vi "PID - Tool.vi"() -> ()   [LabVIEW 2019, in "Control Workspace Tool.lvlib"]
uses:
  Control Workspace Tool.lvlib
  NationalInstruments.VeriStand.SystemStorage
  Types/Tool State Variables.ctl
  Addon/Addon Shared/Types/Get Settings Message.ctl
  Addon/Addon Shared/Types/Gain Schedule.ctl
  <vilib>/NI VeriStand/Execution/Workspace/WorkspaceAPI.ctl
  <vilib>/NI VeriStand/Execution/Workspace/SystemStateRegEventRef.ctl
  <vilib>/NI VeriStand/Execution/Workspace/Target State Info.ctl
  <vilib>/NI VeriStand/Execution/Workspace/Target State.ctl
  <vilib>/NI VeriStand/Execution/Workspace/SystemStateEventRef.ctl
  <vilib>/NI/STM/TCP/TCP Connection Info.ctl
  <vilib>/NI/STM/SubVIs/MetaDataElement.ctl
  Types/UI Refs.ctl
  Workspace Objects/Types/UDP Streaming Command Cluster.ctl
  Workspace Objects/Types/UDP Streaming State.ctl
  Workspace Objects/Types/UI.Chart.Refs.ctl
  Addon/Addon Shared/Types/Update Parameters Message.ctl
  Addon/Addon Shared/SubVIs/Constants.vi
  <vilib>/NI VeriStand/Execution/Workspace/NI VeriStand - Set Single Channel Value.vi
  <vilib>/NI VeriStand/Execution/Workspace/NI VeriStand - Get Multiple Channel Values.vi
  NationalInstruments.VeriStand.SystemDefinitionAPI
  APIs/Host Automation API/Control Host Automation API.lvlib
  Addon/Addon Shared/Control Addon Shared.lvlib
  <vilib>/NI VeriStand/Execution/Workspace/NI_VS Workspace ExecutionAPI.lvlib
  <vilib>/NI/STM/NI STM.lvlib
  Workspace Shared/Control Workspace Shared.lvlib
  Workspace Objects/Control Workspace Object.lvlib
  NationalInstruments.VeriStand.ClientAPI
panel:
  in  "NIVS.Gateway IP Address":string
  out "Gain Scheduling Allowed?":bool
  in  "Revert":bool
  in  "Apply":bool
  out "Live Updates Allowed?":bool
  in  "PID Controller Name":u16(ring) items=["PID Controller", "PID Controller 1"]
  in  "PID Settings":i32(listbox)
  in  "NIVS.System Definition Root":refnum<k24>
  out "Device":string
  in  "NIVS.Workspace Event":refnum<event-registration>
  in  "Hold":bool
  out "Chart":waveform(dbl)[](graph)
  in  "Autoscale Y":bool=TRUE
  in  "Autoscale X":bool=TRUE
  in  "Manual Value":bool
  in  "Setpoint":dbl min=0.0 max=100.0
  in  "Manual Control":bool
  in  "Manual Output":dbl min=0.0 max=100.0
  in  "Revert Control Change":bool
  in  "Apply Control Change":bool
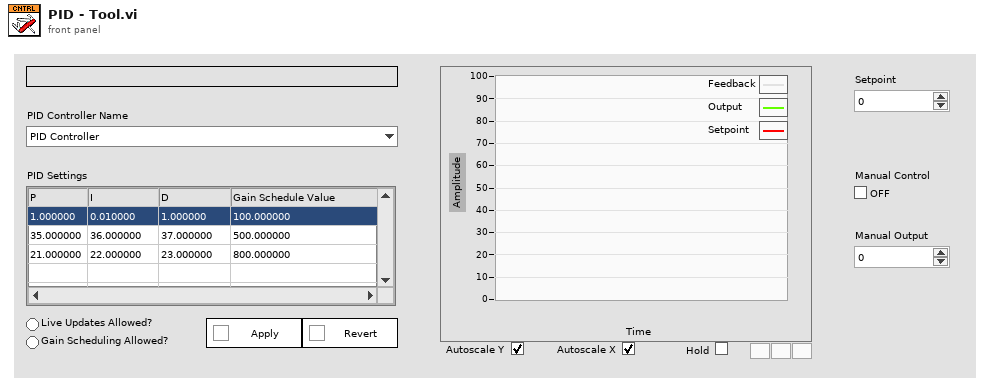
[diagram p1: front panel]
types:
  T1 = typedef "Control Workspace Tool.lvlib/Tool State Variables.ctl" = cluster{"CD Path":string, "CD IP":string, "Settings":T2, "NIVS.SysDefRoot":refnum<k24>, "NIVS.Workspace":T4, "NIVS.UserEvents":cluster{"NIVS.Workspace Event":refnum<event-registration>, "SystemChangeEventRef":T5}, "NIVS.SystemStateRefs":T6, "UI.PIDSettingsMenu":string[], "Comm Info":T7, "Addon.Connected?":bool, "UI.Refs":T9, "NIVS.SysDef":refnum<k24>, "Data.UDPChannels":string[], "Data.Found?":bool, "Data.PreviousValues":dbl[], "Data.SlowChannels":string[], "Data.PendingChange?":bool, "Data.UDPEngineQueue":refnum<queue>, "UI.Chart.Refs":T10, "Controller.SetpointRange":cluster{"Min":dbl, "Max":dbl}, "Controller.OutputRange":cluster{"Min":dbl, "Max":dbl}}
  T2 = typedef "Control Addon Shared.lvlib/Get Settings Message.ctl" = cluster{"Control Loop Names":string[], "Enable Live Updates":bool[], "Gain Schedule":T3[], "Enable Gain Scheduling":bool[]}
  T3 = typedef "Control Addon Shared.lvlib/Gain Schedule.ctl" = cluster{"Gain Schedule":cluster{"PID gains":cluster{"proportional gain (Kc)":dbl, "integral time (Ti, min)":dbl, "derivative time (Td, min)":dbl}, "max value":dbl}[]}
  T4 = typedef "NI_VS Workspace ExecutionAPI.lvlib/WorkspaceAPI.ctl" = refnum<k24>
  T5 = typedef "NI_VS Workspace ExecutionAPI.lvlib/SystemStateRegEventRef.ctl" = refnum<event-registration>
  T6 = typedef "NI_VS Workspace ExecutionAPI.lvlib/SystemStateEventRef.ctl" = cluster{"CustDatRef":refnum<user-event>, "EvtRef":refnum<k27>, "Target State User Event":refnum<user-event>}
  T7 = typedef "NI STM.lvlib/TCP Connection Info.ctl" = cluster{"connection ID":refnum<k5>, "meta data":T8[]}
  T8 = typedef "NI STM.lvlib/MetaDataElement.ctl" = string
  T9 = typedef "Control Workspace Tool.lvlib/UI Refs.ctl" = cluster{"Controller":refnum<vi>, "GainSettings":refnum<vi>, "Device":refnum<vi>, "GainSchedulingAllowed?":refnum<vi>, "LiveUpdatesAllowed?":refnum<vi>, "Revert":refnum<vi>, "Apply":refnum<vi>}
  T10 = typedef "Control Workspace Object.lvlib/UI.Chart.Refs.ctl" = cluster{"Chart":refnum<vi>, "Manual Value":refnum<vi>, "Manual Output":refnum<vi>, "Revert":refnum<vi>, "Apply":refnum<vi>, "Setpoint":refnum<vi>, "Autoscale X":refnum<vi>, "Autoscale Y":refnum<vi>, "Hold":refnum<vi>, "Manual Control":refnum<vi>}
  T11 = typedef "Control Workspace Object.lvlib/UDP Streaming Command Cluster.ctl" = cluster{"Action":T12, "Channels":string[]}
  T12 = typedef "Control Workspace Object.lvlib/UDP Streaming State.ctl" = enum8{"Idle", "Start Acq", "Run", "Stop Acq", "Exit"}
  T13 = typedef "Control Addon Shared.lvlib/Update Parameters Message.ctl" = cluster{"Control Loop":string, "Gain Schedule":cluster{"PID gains":cluster{"proportional gain (Kc)":dbl, "integral time (Ti, min)":dbl, "derivative time (Td, min)":dbl}, "max value":dbl}[]}
  T14 = cluster{"NIVS.Workspace Event":refnum<event-registration>, "SystemChangeEventRef":T5}
  T15 = typedef "LVPoint32TypeDef.ctl" = cluster{"Horizontal":i32, "Vertical":i32}
  T16 = cluster{"PID gains":cluster{"proportional gain (Kc)":dbl, "integral time (Ti, min)":dbl, "derivative time (Td, min)":dbl}, "max value":dbl}[]
  T17 = cluster{"proportional gain (Kc)":dbl, "integral time (Ti, min)":dbl, "derivative time (Td, min)":dbl}
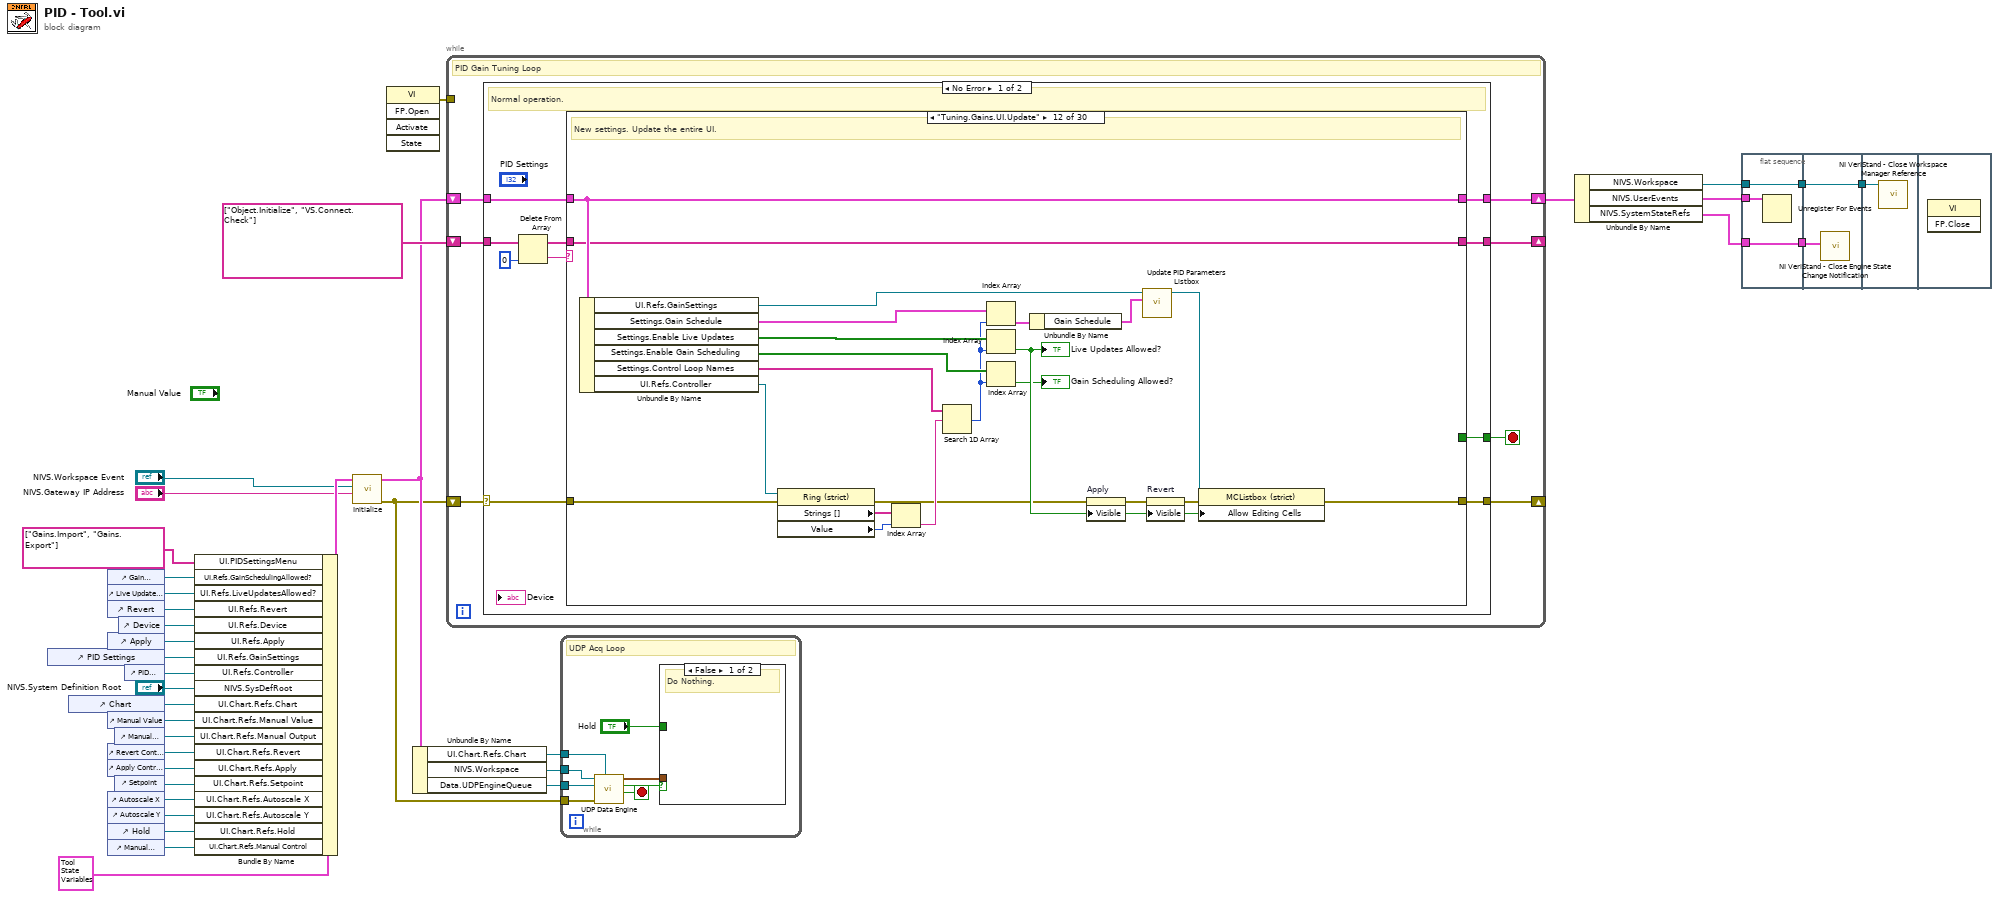
[diagram p0: block diagram]
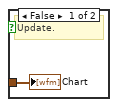
[diagram p3: hidden frame]
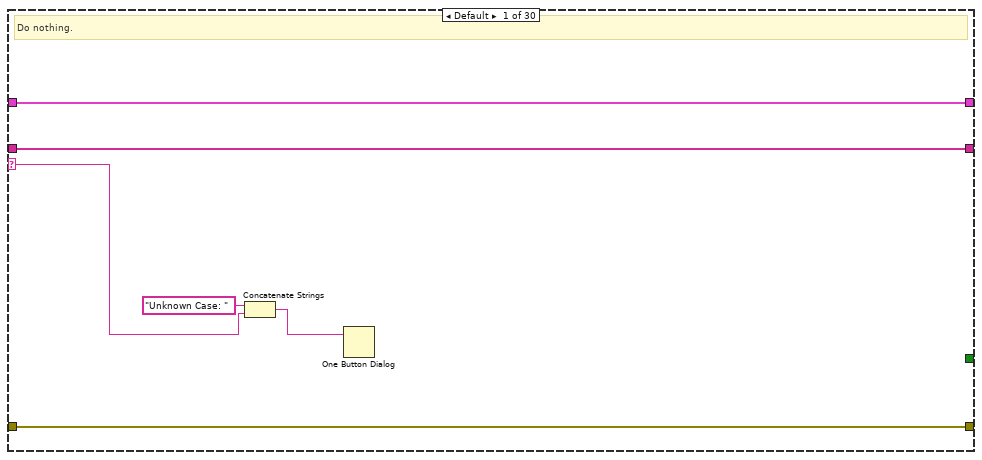
[diagram p4: hidden frame]
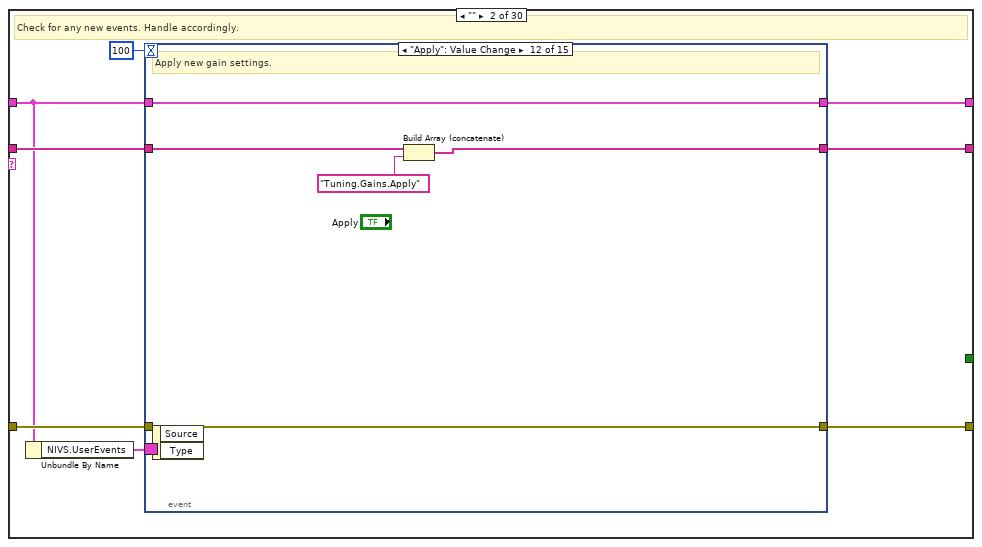
[diagram p5: hidden frame]
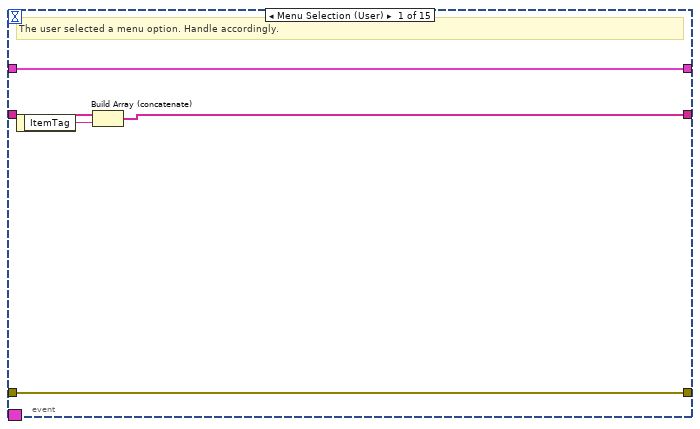
[diagram p6: hidden frame]
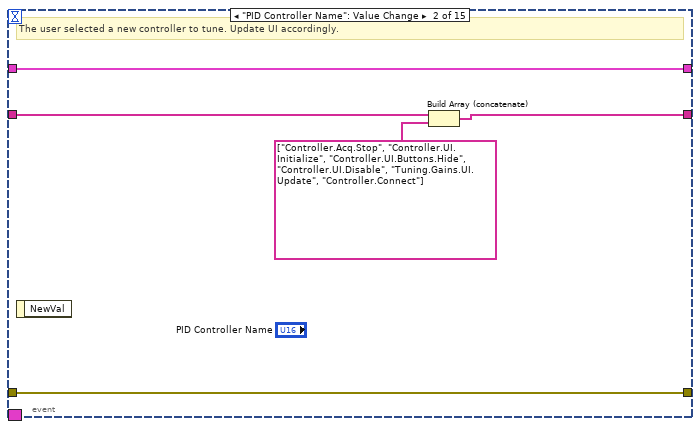
[diagram p7: hidden frame]
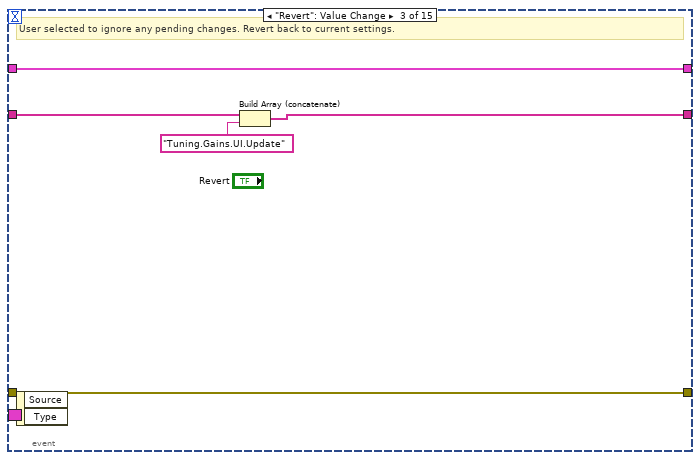
[diagram p8: hidden frame]
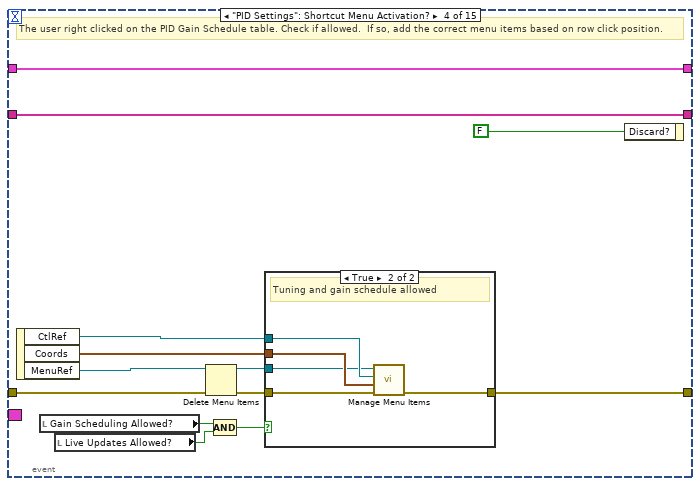
[diagram p9: hidden frame]
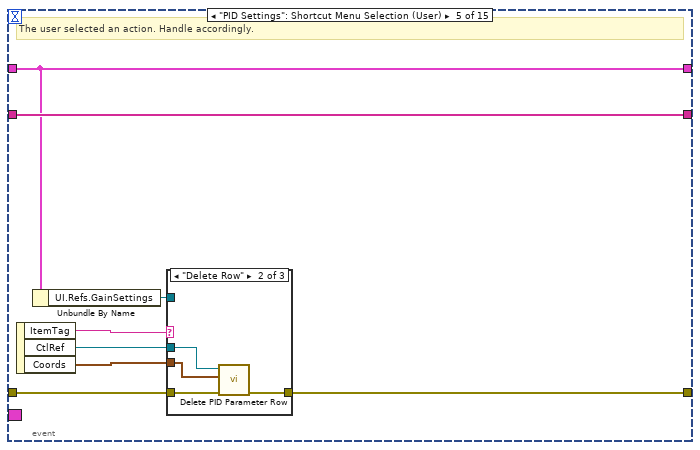
[diagram p11: hidden frame]
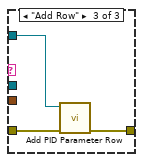
[diagram p13: hidden frame]
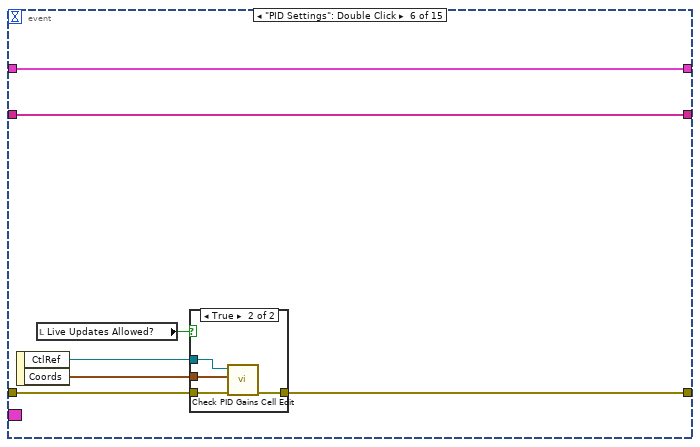
[diagram p14: hidden frame]
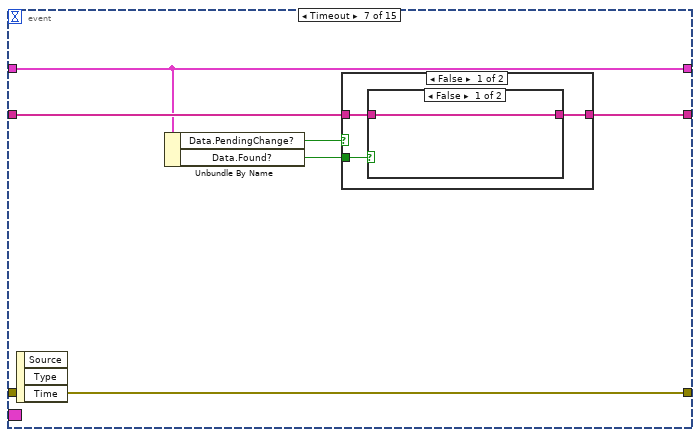
[diagram p16: hidden frame]
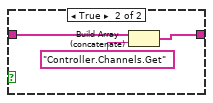
[diagram p17: hidden frame]
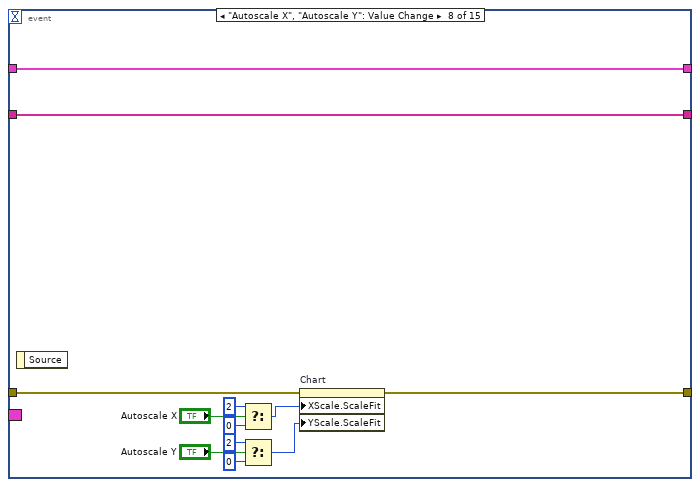
[diagram p19: hidden frame]
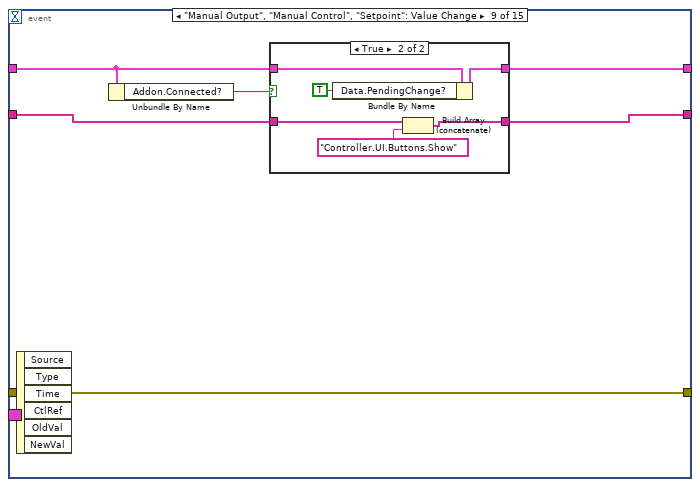
[diagram p20: hidden frame]
diagram:
  n1 = control-ref of="PID Settings"() -> (w32:refnum<vi>)
  n2 = control-ref of="Chart"() -> (w10:refnum<vi>)
  n3 = control-ref of="Gain Scheduling Allowed?"() -> (w24:refnum<vi>)
  n4 = control-ref of="Live Updates Allowed?"() -> (w23:refnum<vi>)
  n5 = control-ref of="Revert"() -> (w22:refnum<vi>)
  n6 = control-ref of="Apply"() -> (w21:refnum<vi>)
  n7 = control-ref of="Manual Value"() -> (w2:refnum<vi>)
  n8 = control-ref of="Revert Control Change"() -> (w9:refnum<vi>)
  n9 = control-ref of="Apply Control Change"() -> (w8:refnum<vi>)
  n10 = control-ref of="Autoscale X"() -> (w6:refnum<vi>)
  n11 = control-ref of="Autoscale Y"() -> (w5:refnum<vi>)
  n12 = control-ref of="Hold"() -> (w4:refnum<vi>)
  n13 = control-ref of="Manual Control"() -> (w3:refnum<vi>)
  n14 = control-ref of="Manual Output"() -> (w1:refnum<vi>)
  n15 = control-ref of="Setpoint"() -> (w7:refnum<vi>)
  n16 = control-ref of="Device"() -> (w20:refnum<vi>)
  n17 = control-ref of="PID Controller Name"() -> (w31:refnum<vi>)
  n18 = Bundle By Name(cluster=T1 {"CD Path"="", "CD IP"="", "Settings"={"Control Loop Names"=[], "Enable Live Updates"=[], "Gain Schedule"=[], "Enable Gain Scheduling"=[]}, "NIVS.SysDefRoot"=refnum, "NIVS.Workspace"=refnum, "NIVS.UserEvents"={"NIVS.Workspace Event"=refnum, "SystemChangeEventRef"=refnum}, "NIVS.SystemStateRefs"={"CustDatRef"=refnum, "EvtRef"=refnum, "Target State User Event"=refnum}, "UI.PIDSettingsMenu"=[], "Comm Info"={"connection ID"=refnum, "meta data"=[]}, "Addon.Connected?"=FALSE, "UI.Refs"={"Controller"=refnum, "GainSettings"=refnum, "Device"=refnum, "GainSchedulingAllowed?"=refnum, "LiveUpdatesAllowed?"=refnum, "Revert"=refnum, "Apply"=refnum}, "NIVS.SysDef"=refnum, "Data.UDPChannels"=[], "Data.Found?"=FALSE, "Data.PreviousValues"=[], "Data.SlowChannels"=[], "Data.PendingChange?"=FALSE, "Data.UDPEngineQueue"=refnum, "UI.Chart.Refs"={"Chart"=refnum, "Manual Value"=refnum, "Manual Output"=refnum, "Revert"=refnum, "Apply"=refnum, "Setpoint"=refnum, "Autoscale X"=refnum, "Autoscale Y"=refnum, "Hold"=refnum, "Manual Control"=refnum}, "Controller.SetpointRange"={"Min"=0.0, "Max"=0.0}, "Controller.OutputRange"={"Min"=0.0, "Max"=0.0}}, "UI.PIDSettingsMenu"=string[] ["Gains.Import", "Gains.Export"], "UI.Refs.GainSchedulingAllowed?"=w24, "UI.Refs.LiveUpdatesAllowed?"=w23, "UI.Refs.Revert"=w22, "UI.Refs.Device"=w20, "UI.Refs.Apply"=w21, "UI.Refs.GainSettings"=w32, "UI.Refs.Controller"=w31, "NIVS.SysDefRoot"="NIVS.System Definition Root", "UI.Chart.Refs.Chart"=w10, "UI.Chart.Refs.Manual Value"=w2, "UI.Chart.Refs.Manual Output"=w1, "UI.Chart.Refs.Revert"=w9, "UI.Chart.Refs.Apply"=w8, "UI.Chart.Refs.Setpoint"=w7, "UI.Chart.Refs.Autoscale X"=w6, "UI.Chart.Refs.Autoscale Y"=w5, "UI.Chart.Refs.Hold"=w4, "UI.Chart.Refs.Manual Control"=w3) -> (w15:T1)
  n19 = call "Initialize.vi"("NIVS.Gateway IP Address"="NIVS.Gateway IP Address", "NIVS.Workspace Event"="NIVS.Workspace Event", "State Variables"=w15) -> ("error out"=w11:errorcluster, "output cluster"=w12:T1)  [unwired: 7 in]
  n20 = invoke class="VI" method="FP.Open"() -> (error out=w36:errorcluster)  [unwired: 5 in, 4 out]
  n21 = Unbundle By Name(w12) -> ("UI.Chart.Refs.Chart"=w19:refnum<vi>, "NIVS.Workspace"=w18:T4, "Data.UDPEngineQueue"=w17:refnum<queue>)
  n22 = while {
    shift-right: [w42] -> w29
    shift-left: w12 -> [w43]
    shift-right: [w40] -> _
    shift-left: string[] ["Object.Initialize", "VS.Connect.Check"] -> [w41]
    tunnel: w36 -> [_]
    shift-right: [w39] -> _
    shift-left: w11 -> [w38]
    stop <- w44 stop-if-true
    # "PID Gain Tuning Loop"
    n23 = case shown="No Error" w38 {
      selector: w38 -> [w45 w764]
      tunnel: [w54 _] -> w44
      tunnel: w43 -> [w53 w766]
      tunnel: [w52 w766] -> w42
      tunnel: w41 -> [w51 w765]
      tunnel: [w47 w765] -> w40
      tunnel: [w46 w762] -> w39
      frame No Error {
        # "Normal operation."
        n24 = Delete From Array(array=w51, index=0) -> (deleted portion=w49:string, array with subset deleted=w48:string[])  [unwired: 1 in]
        n25 = case shown="\"Tuning.Gains.UI.Update\"" w49 {
          selector: w49 -> [w57 _ _ _ _ _ _ _ _ _ _ _ _ _ _ _ _ _ _ _ _ _ _ _ _ _ _ _ _ _]
          tunnel: [_ _ _ _ _ _ _ TRUE ("Discard?") _ _ _ _ _ _ _ _ _ _ _ _ _ _ _ _ _ _ _ _ _ _] -> w54
          tunnel: w53 -> [w59 w63 w223 w251 w268 w277 w296 w314 w319 w330 w338 w367 w370 w411 w440 w494 w512 w525 w538 w552 w573 w581 w625 w679 w702 w724 w732 w744 w752 w756]
          tunnel: [w59 w68 w224 w246 w268 w278 w297 w313 w319 w331 w339 w367 w370 w411 w448 w493 w512 w525 w538 w551 w573 w582 w626 w680 w703 w725 w733 w744 w747 w755] -> w52
          tunnel: w48 -> [w60 w67 w222 w245 w266 w280 w299 w316 w318 w337 w345 w346 w373 w413 w446 w490 w516 w527 w533 w555 w580 w599 w637 w691 w723 w731 w739 w745 w753 w761]
          tunnel: [w60 w66 w221 w244 w267 w279 w298 w316 w318 w337 w345 w346 w372 w413 w445 w489 w516 w527 w533 w556 w580 w599 w637 w691 w723 w731 w739 w745 w753 w761] -> w47
          tunnel: [w58 w64 w225 w241 w264 w272 w290 w305 w320 w334 w342 w347 w368 w412 w441 w487 w513 w522 w535 w557 w574 w584 w624 w672 w709 w728 w736 w740 w748 w757] -> w46
          tunnel: w45 -> [w58 w65 w233 w240 w264 w281 w300 w306 w324 w335 w343 w352 w369 w410 w438 w487 w514 w523 w536 w548 w575 w583 w627 w677 w697 w729 w737 w741 w749 w758]
          frame Default {
            # "Do nothing."
            n26 = Concatenate Strings("Unknown Case: " ("string"), w57) -> (w56:string)
            n27 = One Button Dialog(message=w56) -> ()  [unwired: 1 in, 1 out]
          }
          frame "" {
            # "Check for any new events. Handle accordingly."
            n28 = Unbundle By Name(w63) -> ("NIVS.UserEvents"=w62:T14)
            n29 = event shown="[11] \"Apply\": Value Change" {
              selector: w62 -> [_ _ _ _ _ _ _ _ _ _ _ _ _ _ _]
              dyn-events: _ -> [_ _ _ _ _ _ _ _ _ _ _ _ _ _ _]
              timeout: 100 -> [_ _ _ _ _ _ _ _ _ _ _ _ _ _ _]
              tunnel: w63 -> [w71 w77 w83 w90 w104 w125 w133 w156 w157 w175 w176 w184 w197 w203 w217]
              tunnel: [w71 w77 w83 w90 w104 w125 w133 w156 w158 w175 w177 w184 w197 w203 w217] -> w68
              tunnel: w67 -> [w73 w76 w82 w96 w110 w124 w135 w155 w159 w172 w178 w187 w196 w206 w215]
              tunnel: [w70 w74 w81 w96 w110 w124 w134 w155 w160 w171 w179 w186 w195 w205 w214] -> w66
              tunnel: w65 -> [w69 w78 w79 w86 w106 w123 w136 w145 w162 w174 w182 w183 w194 w204 w213]
              tunnel: [w69 w78 w79 w85 w105 w122 w136 w146 w162 w174 w182 w183 w194 w204 w213] -> w64
              event Menu Selection (User) {
                # "The user selected a menu option. Handle accordingly."
                n30 = event-data() -> ("ItemTag"=w72:string)  [unwired: 1 out]
                n31 = Build Array (concatenate)(w73, w72) -> (w70:string[])
              }
              event "PID Controller Name": Value Change {
                # "The user selected a new controller to tune. Update UI accordingly."
                n32 = event-data() -> ()  [unwired: 2 out]
                n33 = Build Array (concatenate)(w76, string[] ["Controller.Acq.Stop", "Controller.UI.Initialize", "Controller.UI.Buttons.Hide", "Controller.UI.Disable", "Tuning.Gains.UI.Update", "Controller.Connect"]) -> (w74:string[])
              }
              event "Revert": Value Change {
                # "User selected to ignore any pending changes. Revert back to current settings."
                n34 = event-data() -> ()  [unwired: 3 out]
                n35 = Build Array (concatenate)(w82, "Tuning.Gains.UI.Update") -> (w81:string[])
              }
              event "PID Settings": Shortcut Menu Activation? {
                # "The user right clicked on the PID Gain Schedule table. Check if allowed.  If so, add the correct menu items based on row click position."
                n36 = event-data() -> ("CtlRef"=w93:refnum<vi>, "Coords"=w92:T15, "MenuRef"=w84:refnum<k9>)  [unwired: 1 out]
                n37 = local read "Gain Scheduling Allowed?"() -> (w89:bool)
                n38 = local read "Live Updates Allowed?"() -> (w87:bool)
                n39 = Delete Menu Items(6:w86, 9:w84) -> (0:w94:errorcluster, 3:w95:refnum<k9>)  [unwired: 2 in]
                n40 = Compound Arithmetic op=AND(w89, w87) -> (w88:bool)
                n41 = case shown="True" w88 {
                  tunnel: w93 -> [_ w102]
                  tunnel: w92 -> [_ w101]
                  tunnel: w95 -> [_ w100]
                  tunnel: [w97 w99] -> w85
                  tunnel: w94 -> [w97 w98]
                  frame False {
                    # "Tuning or gain schedule not allowed"
                  }
                  frame True {
                    # "Tuning and gain schedule allowed"
                    n42 = call "Manage Menu Items.vi"("error in (no error)"=w98, "Coords"=w101, "CtlRef"=w102, "Menu in"=w100) -> ("error out"=w99:errorcluster)  [unwired: 7 in]
                  }
                }
                n43 = event-data("Discard?"=FALSE) -> ()  [unwired: 1 in, 1 out]
              }
              event "PID Settings": Shortcut Menu Selection (User) {
                # "The user selected an action. Handle accordingly."
                n44 = event-data() -> ("ItemTag"=w107:string, "CtlRef"=w108:refnum<vi>, "Coords"=w109:T15)  [unwired: 1 out]
                n45 = Unbundle By Name(w104) -> ("UI.Refs.GainSettings"=w103:refnum<vi>)
                n46 = case shown="\"Delete Row\"" w107 {
                  tunnel: w103 -> [_ _ w118]
                  tunnel: [w111 w113 w117] -> w105
                  tunnel: w108 -> [_ w115 _]
                  tunnel: w109 -> [_ w114 _]
                  tunnel: w106 -> [w111 w112 w116]
                  frame Default {
                  }
                  frame "Delete Row" {
                    n47 = call "Delete PID Parameter Row.vi"("error in (no error)"=w112, "Coords"=w114, "MulticolumnListbox in"=w115) -> ("error out"=w113:errorcluster)  [unwired: 8 in]
                  }
                  frame "Add Row" {
                    n48 = call "Add PID Parameter Row.vi"("error in (no error)"=w116, "MulticolumnListbox in"=w118) -> ("error out"=w117:errorcluster)  [unwired: 9 in]
                  }
                }
              }
              event "PID Settings": Double Click {
                n49 = event-data() -> ("CtlRef"=w121:refnum<vi>, "Coords"=w120:T15)  [unwired: 1 out]
                n50 = local read "Live Updates Allowed?"() -> (w119:bool)
                n51 = case shown="True" w119 {
                  tunnel: w123 -> [w126 w130]
                  tunnel: [w126 w129] -> w122
                  tunnel: w121 -> [_ w128]
                  tunnel: w120 -> [_ w127]
                  frame False {
                  }
                  frame True {
                    n52 = call "Check PID Gains Cell Edit.vi"("error in (no error)"=w130, "Coords"=w127, "MulticolumnListbox in"=w128) -> ("error out"=w129:errorcluster)  [unwired: 8 in]
                  }
                }
              }
              event Timeout {
                n53 = event-data() -> ()  [unwired: 4 out]
                n54 = Unbundle By Name(w133) -> ("Data.PendingChange?"=w132:bool, "Data.Found?"=w131:bool)
                n55 = case shown="False" w132 {
                  tunnel: w135 -> [w139 w144]
                  tunnel: [w138 w144] -> w134
                  tunnel: w131 -> [w137 _]
                  frame False {
                    n56 = case shown="False" w137 {
                      tunnel: w139 -> [w140 w142]
                      tunnel: [w140 w141] -> w138
                      frame False {
                      }
                      frame True {
                        n57 = Build Array (concatenate)(w142, "Controller.Channels.Get") -> (w141:string[])
                      }
                    }
                  }
                  frame True {
                  }
                }
              }
              event "Autoscale X", "Autoscale Y": Value Change {
                n58 = event-data() -> ()  [unwired: 2 out]
                n59 = Select(t=u8 2, s="Autoscale X", f=u8 0 ("X Scale.Scale Fit")) -> (s? t:f=w152:u8)
                n60 = Select(t=u8 2, s="Autoscale Y", f=u8 0 ("X Scale.Scale Fit")) -> (s? t:f=w154:u8)
                n61 = property on="Chart" class="WFChart (strict)"(error in=w145, "XScale.ScaleFit"=w152, "YScale.ScaleFit"=w154) -> (error out=w146:errorcluster)  [unwired: 1 in, 1 out]
              }
              event "Manual Output", "Manual Control", "Setpoint": Value Change {
                n62 = event-data() -> ()  [unwired: 7 out]
                n63 = Unbundle By Name(w157) -> ("Addon.Connected?"=w161:bool)
                n64 = case shown="True" w161 {
                  tunnel: w157 -> [w163 w169]
                  tunnel: [w163 w168] -> w158
                  tunnel: w159 -> [w164 w167]
                  tunnel: [w164 w165] -> w160
                  frame False {
                  }
                  frame True {
                    n65 = Bundle By Name(cluster=w169, "Data.PendingChange?"=TRUE ("Pending Change?")) -> (w168:T1)
                    n66 = Build Array (concatenate)(w167, "Controller.UI.Buttons.Show") -> (w165:string[])
                  }
                }
              }
              event "Apply Control Change": Value Change {
                n67 = event-data() -> ()  [unwired: 2 out]
                n68 = Build Array (concatenate)(w172, string[] ["Controller.Channels.Set", "Controller.UI.Buttons.Hide"]) -> (w171:string[])
              }
              event "Revert Control Change": Value Change {
                n69 = event-data() -> ()  [unwired: 2 out]
                n70 = Bundle By Name(cluster=w176, "Data.PendingChange?"=FALSE ("Pending Change?")) -> (w177:T1)
                n71 = Build Array (concatenate)(w178, string[] ["Controller.Channels.Get", "Controller.UI.Buttons.Hide"]) -> (w179:string[])
              }
              event "Apply": Value Change {
                # "Apply new gain settings."
                n72 = event-data() -> ()  [unwired: 3 out]
                n73 = Build Array (concatenate)(w187, "Tuning.Gains.Apply") -> (w186:string[])
              }
              event User Event {
                # "A workspace event occurred. Handle accordingly."
                n74 = event-data() -> ("Workspace Event"=w189:string)  [unwired: 1 out]
                n75 = Equal?(x=w189, y="Shut Down") -> (x = y?=w190:bool)
                n76 = Equal?(x=w189, y="Disconnect") -> (x = y?=w191:bool)
                n77 = Compound Arithmetic op=OR(w190, w191) -> (w188:bool)
                n78 = case shown="True" w188 {
                  tunnel: w196 -> [w198 w201]
                  tunnel: [w198 w199] -> w195
                  frame False {
                  }
                  frame True {
                    n79 = Build Array (concatenate)(w201, "Object.Exit" ("y")) -> (w199:string[])
                  }
                }
              }
              event User Event {
                # "The system state changed. Handle accordingly."
                n80 = event-data() -> ("SystemStateChange"=w202:string)  [unwired: 1 out]
                n81 = case shown="Default" w202 {
                  tunnel: w206 -> [w209 w212]
                  tunnel: [w208 w211] -> w205
                  frame "Stop Configuration" {
                    # "Not connected"
                    n82 = Build Array (concatenate)(w209, "Object.Exit") -> (w208:string[])
                  }
                  frame Default {
                    # "Connected"
                    n83 = Build Array (concatenate)(w212, "VS.Connect.Check") -> (w211:string[])
                  }
                }
              }
              event Panel Close? {
                # "The user attempted to close the panel. Discard this event and handle it in a controlled way."
                n84 = event-data() -> ()  [unwired: 5 out]
                n85 = Build Array (concatenate)(w215, "Object.Exit" ("y")) -> (w214:string[])
                n86 = event-data("Discard?"=TRUE) -> ()  [unwired: 1 in, 1 out]
              }
            }
          }
          frame "VS.Connect.Check" {
            n87 = Unbundle By Name(w223) -> ("UI.Refs.Device"=w229:refnum<vi>, "NIVS.Workspace"=w231:T4, "NIVS.SysDefRoot"=w232:refnum<k24>, "CD Path"=w230:string)
            n88 = Current VI's Menubar() -> (w228:refnum<k9>)
            n89 = call "UI.Connection.State.Get.vi"("Menu Ref"=w228, "Name Ref"=w229, "error in (no error)"=w233, "Addon Path in"=w230, "NIVS.System Definition Root in"=w232, "NIVS.Workspace Ref in"=w231) -> ("error out"=w225:errorcluster, "Addon Connected?"=w220:bool, "NIVS.System Definition Root out"=w226:refnum<k24>, "NIVS.Workspace Ref out"=w227:T4, "NIVS.SysDef Ref out"=w219:refnum<k24>)  [unwired: 1 in]
            n90 = Bundle By Name(cluster=w223, "NIVS.SysDef"=w219, "NIVS.Workspace"=w227, "NIVS.SysDefRoot"=w226, "Addon.Connected?"=w220) -> (w224:T1)
            n91 = case shown="True" w220 {
              tunnel: [w235 w238] -> w221
              tunnel: w222 -> [w236 w239]
              frame True {
                n92 = Build Array (concatenate)(w236, "Object.Connected") -> (w235:string[])
              }
              frame False {
                n93 = Build Array (concatenate)(w239, "Object.Disconnected") -> (w238:string[])
              }
            }
          }
          frame "Object.Configure" {
            # "User selected to configure which control addon instance is selected. Popup addon selection dialog. Connect based on selection."
            n94 = Unbundle By Name(w251) -> ("NIVS.SysDefRoot"=w243:refnum<k24>, "CD Path"=w250:string)
            n95 = global read "Constants.vi" "GUID.Control"() -> (w242:string)
            n96 = call "Select Custom Device.vi"("Main GUID"=w242, "CD Path"=w250, "NIVS.System Definition Root"=w243) -> ("Cancelled?"=w249:bool, "IP Address"=w248:string, "Custom Device Path Out"=w247:string)  [unwired: 6 in]
            n97 = case shown="False" w249 {
              tunnel: w248 -> [w256 _]
              tunnel: w247 -> [w257 _]
              tunnel: w251 -> [w254 w263]
              tunnel: [w255 w263] -> w246
              tunnel: w245 -> [w260 w262]
              tunnel: [w259 w262] -> w244
              tunnel: [w258 w261] -> w241
              tunnel: w240 -> [w258 w261]
              frame False {
                w252 = FALSE ("Data.PendingChange?")
                # "Addon selected."
                n98 = Bundle By Name(cluster=w254, "CD Path"=w257, "CD IP"=w256, "Data.PendingChange?"=w252, "Data.Found?"=w252) -> (w255:T1)
                n99 = Build Array (concatenate)(w260, string[] ["Object.Initialize", "VS.Connect.Check"]) -> (w259:string[])
              }
              frame True {
                # "User canceled."
              }
            }
          }
          frame "Object.Initialize" {
            # "Initialize the tool UI, buttons, and check current system state."
            n100 = Build Array (concatenate)(w266, string[] ["Tuning.UI.Initialize", "Tuning.Gains.Menu.Disable", "Tuning.UI.Disable", "Controller.UI.Initialize", "Controller.UI.Buttons.Hide", "Controller.UI.Disable", "Controller.Acq.Stop"]) -> (w267:string[])
          }
          frame "Object.Connected" {
            n101 = Unbundle By Name(w277) -> ("CD Path"=w269:string, "CD IP"=w274:string, "Comm Info"=w273:T7)
            n102 = call "Close Connection with CD.vi"("error in"=w281, "connection info"=w273) -> ("error out"=w276:errorcluster)  [unwired: 9 in]
            n103 = flat-sequence {
              tunnel: w274 -> [w287]
              tunnel: w269 -> [w288]
              tunnel: [w285] -> w270
              tunnel: w276 -> [_]
              tunnel: [w286] -> w275
              frame #0 {
                n104 = call "Check Network Connection.vi"("IP Address"=w287, "CD Path"=w288) -> ("error out"=w285:errorcluster, "connection info"=w286:T7)  [unwired: 8 in]
              }
            }
            n105 = case shown="No Error" w270 {
              selector: w270 -> [w282 w284]
              tunnel: [w282 w284] -> w272
              tunnel: [string[] ["Tuning.Gains.Connect"] _] -> w271
              frame No Error {
              }
              frame Error {
              }
            }
            n106 = Build Array (concatenate)(w280, w271) -> (w279:string[])
            n107 = Bundle By Name(cluster=w277, "CD Path"=w269, "CD IP"=w274, "Comm Info"=w275) -> (w278:T1)
          }
          frame "Object.Disconnected" {
            n108 = Unbundle By Name(w296) -> ("CD Path"=w295:string, "CD IP"=w294:string, "Comm Info"=w293:T7, "UI.Refs"=w289:T9)
            n109 = flat-sequence {
              tunnel: w300 -> [w302]
              tunnel: w293 -> [w303]
              tunnel: [w302] -> w290
              tunnel: [w301] -> _
              frame #0 {
                n110 = call "Close Connection with CD.vi"("error in"=w302, "connection info"=w303) -> ("error out"=w301:errorcluster)  [unwired: 9 in]
              }
            }
            n111 = Bundle By Name(cluster=w296, "CD Path"=w295, "CD IP"=w294, "Comm Info"=T7 {"connection ID"=refnum, "meta data"=[]} ("connection info"), "UI.Refs"=w289) -> (w297:T1)
            n112 = Build Array (concatenate)(w299, string[] ["Object.Initialize"]) -> (w298:string[])
          }
          frame "Object.Exit" {
            # "Exit the tool. Kill the custom device communication reference."
            n113 = Unbundle By Name(w314) -> ("Comm Info"=w312:T7, "Data.UDPEngineQueue"=w304:refnum<queue>)
            n114 = call "Close Connection with CD.vi"("connection info"=w312) -> ()  [unwired: 10 in, 1 out]
            n115 = Enqueue Element(queue=w304, element=T11 {"Action"=enum."Stop Acq", "Channels"=[]}, error in (no error)=w306) -> (queue out=w309:refnum<queue>, error out=w307:errorcluster)  [unwired: 1 in, 1 out]
            n116 = Bundle By Name(cluster=w314, "Comm Info"=T7 {"connection ID"=refnum, "meta data"=[]} ("connection info")) -> (w313:T1)
            n117 = Enqueue Element(queue=w309, element=T11 {"Action"=enum."Exit", "Channels"=[]}, error in (no error)=w307) -> (error out=w305:errorcluster)  [unwired: 1 in, 2 out]
          }
          frame "Tuning.UI.Initialize" {
            w323 = FALSE ("Allow Editing Cells")
            # "Initialize the tool UI, buttons, and check current system state."
            n118 = Unbundle By Name(w319) -> ("UI.Refs.GainSettings"=w321:refnum<vi>, "UI.Refs.Controller"=w322:refnum<vi>)
            n119 = property class="Ring (strict)"(reference=w322, error in=w324, "Strings []"=string[] [], "Value"=u16 0) -> (error out=w329:errorcluster)  [unwired: 1 out]
            n120 = local write "Gain Scheduling Allowed?"(w323) -> ()
            n121 = local write "Live Updates Allowed?"(w323) -> ()
            n122 = property class="MCListbox (strict)"(reference=w321, error in=w329, "ItemNames"=string[][] [] ("Item Names"), "Allow Editing Cells"=w323) -> (error out=w325:errorcluster)  [unwired: 1 out]
            n123 = property on="Apply" class="Bool"(error in=w325, "Visible"=w323) -> (error out=w326:errorcluster)  [unwired: 1 in, 1 out]
            n124 = property on="Revert" class="Bool"(error in=w326, "Visible"=w323) -> (error out=w320:errorcluster)  [unwired: 1 in, 1 out]
          }
          frame "Tuning.UI.Enable" {
            n125 = Unbundle By Name(w330) -> ("UI.Refs"=w333:T9)
            n126 = call "UI Set DisableState.vi"("Enable?"=TRUE, "error in (no error)"=w335, "UI.Refs"=w333) -> ("error out"=w334:errorcluster, "UI.Refs out"=w332:T9)  [unwired: 7 in]
            n127 = Bundle By Name(cluster=w330, "UI.Refs"=w332) -> (w331:T1)
          }
          frame "Tuning.UI.Disable" {
            n128 = Unbundle By Name(w338) -> ("UI.Refs"=w341:T9)
            n129 = call "UI Set DisableState.vi"("Enable?"=FALSE, "error in (no error)"=w343, "UI.Refs"=w341) -> ("error out"=w342:errorcluster, "UI.Refs out"=w340:T9)  [unwired: 7 in]
            n130 = Bundle By Name(cluster=w338, "UI.Refs"=w340) -> (w339:T1)
          }
          frame "Tuning.Gains.UI.Update" {
            # "New settings. Update the entire UI."
            n131 = Unbundle By Name(w367) -> ("UI.Refs.GainSettings"=w350:refnum<vi>, "Settings.Gain Schedule"=w360:T3[], "Settings.Enable Live Updates"=w365:bool[], "Settings.Enable Gain Scheduling"=w355:bool[], "Settings.Control Loop Names"=w358:string[], "UI.Refs.Controller"=w351:refnum<vi>)
            n132 = property class="Ring (strict)"(reference=w351, error in=w352) -> (error out=w349:errorcluster, "Strings []"=w363:string[], "Value"=w362:u16)  [unwired: 1 out]
            n133 = Index Array(array=w363, index=w362) -> (element=w366:string)
            n134 = Search 1D Array(1D array=w358, element=w366) -> (index of element=w354:i32)  [unwired: 1 in]
            n135 = Index Array(array=w360, index=w354) -> (element=w359:T3)
            n136 = Index Array(array=w365, index=w354) -> (element=w356:bool)
            "Live Updates Allowed?" <- w356
            n137 = Index Array(array=w355, index=w354) -> (element=→"Gain Scheduling Allowed?":bool)
            n138 = Unbundle By Name(w359) -> ("Gain Schedule"=w361:T16)
            n139 = property on="Apply" class="Bool"(error in=w349, "Visible"=w356) -> (error out=w364:errorcluster)  [unwired: 1 in, 1 out]
            n140 = call "Update PID Parameters Listbox.vi"("Gain Schedule"=w361, "MulticolumnListbox in"=w350) -> ("MulticolumnListbox out"=w357:refnum<vi>)  [unwired: 9 in]
            n141 = property on="Revert" class="Bool"(error in=w364, "Visible"=w356) -> (error out=w348:errorcluster)  [unwired: 1 in, 1 out]
            n142 = property class="MCListbox (strict)"(reference=w357, error in=w348, "Allow Editing Cells"=w356) -> (error out=w347:errorcluster)  [unwired: 1 out]
          }
          frame "Tuning.Gains.Import" {
            # "Import gains settings for the current controller from disk. Load as temporary settings but ask user if they want to apply them."
            n143 = call "Import PID Parameters.vi"("error in"=w369) -> ("error out"=w371:errorcluster, "Apply?"=w375:bool, "Parameters"=w374:dbl[][])  [unwired: 8 in]
            n144 = case shown="True" w375 {
              tunnel: w374 -> [_ w384]
              tunnel: w373 -> [w377 w382]
              tunnel: [w377 w383] -> w372
              tunnel: w371 -> [w376 w378]
              tunnel: w370 -> [_ w381]
              tunnel: [w376 w379] -> w368
              frame False {
                # "Import failed."
              }
              frame True {
                # "Settings import successful. Apply and ask user if they want to apply these temp settings."
                n145 = for {
                  tunnel: w384 -> [w402] mode=indexing
                  tunnel: [w401] -> w387 mode=indexing
                  tunnel: [w400] -> w385 mode=indexing
                  tunnel: w378 -> [w398]
                  n146 = for {
                    tunnel: w402 -> [w404] mode=indexing
                    tunnel: [w406] -> w401 mode=indexing
                    tunnel: [w405] -> w399 mode=indexing
                    tunnel: w398 -> [w403]
                    n147 = Format Into String(error in=w403, w404) -> (resulting string=w406:string, error out=w405:errorcluster)  [unwired: 2 in]
                  }
                  n148 = Merge Errors(w399) -> (w400:errorcluster)
                }
                n149 = Unbundle By Name(w381) -> ("UI.Refs.GainSettings"=w380:refnum<vi>)
                n150 = Merge Errors(w385) -> (w386:errorcluster)
                n151 = property class="MCListbox (strict)"(reference=w380, error in=w386, "ItemNames"=w387) -> (error out=w379:errorcluster)  [unwired: 1 out]
                n152 = flat-sequence {
                  tunnel: [w393] -> w383
                  tunnel: w382 -> [w392]
                  tunnel: w379 -> [_]
                  frame #0 {
                    n153 = Two Button Dialog(message="Would you like to apply the imported values?", 1:"No" ("F button name (\"Cancel\")"), 2:"Yes" ("T button name (\"OK\")")) -> (T button?=w390:bool)
                    n154 = case shown="True" w390 {
                      tunnel: [w394 w397] -> w393
                      tunnel: w392 -> [w394 w396]
                      frame False {
                      }
                      frame True {
                        n155 = Build Array (concatenate)(w396, "Gains.Apply") -> (w397:string[])
                      }
                    }
                  }
                }
              }
            }
          }
          frame "Tuning.Gains.Export" {
            # "Export the current gain settings for the current controller to disk."
            n156 = Unbundle By Name(w411) -> ("UI.Refs.GainSettings"=w407:refnum<vi>, "UI.Refs.Controller"=w408:refnum<vi>)
            n157 = property class="Ring (strict)"(reference=w408, error in=w410) -> (error out=w409:errorcluster, "Strings []"=w416:string[], "Value"=w417:u16)  [unwired: 1 out]
            n158 = call "Get and Check PID Parameters.vi"("error in (no error)"=w409, "MulticolumnListbox in"=w407) -> ("error out"=w418:errorcluster, "PID Parameters"=w415:T16, "MulticolumnListbox out"=w414:refnum<vi>)  [unwired: 7 in]
            n159 = Index Array(array=w416, index=w417) -> (element=w419:string)
            n160 = case shown="No Error" w418 {
              selector: w418 -> [_ w430]
              tunnel: w419 -> [w423 _]
              tunnel: w414 -> [_ _]
              tunnel: w415 -> [w422 _]
              tunnel: [w420 w429] -> w412
              frame No Error {
                n161 = for {
                  tunnel: w422 -> [w428] mode=indexing
                  tunnel: [w424] -> w421 mode=indexing
                  n162 = Unbundle By Name(w428) -> ("PID gains"=w427:T17, "max value"=w425:dbl)
                  n163 = Cluster To Array(cluster=w427) -> (array=w426:dbl[])
                  n164 = Build Array (concatenate)(w426, w425) -> (w424:dbl[])
                }
                n165 = call "Export PID Parameters.vi"("Parameters"=w421, "Control Loop"=w423) -> ("error out"=w420:errorcluster)  [unwired: 9 in]
              }
              frame Error {
                n166 = call <vilib>:"Clear Errors.vi"("error in (no error)"=w430) -> ("error out"=w429:errorcluster)  [unwired: 5 in, 1 out]
              }
            }
          }
          frame "Tuning.Gains.Apply" {
            # "User selected to apply updates. Get the current controller & settings, make sure settings are valid, connect to the addon, apply settings, handle errors."
            n167 = Unbundle By Name(w440) -> ("NIVS.SysDef"=w431:refnum<k24>, "NIVS.SysDefRoot"=w432:refnum<k24>, "Comm Info"=w433:T7, "CD Path"=w435:string, "CD IP"=w434:string, "UI.Refs.GainSettings"=w436:refnum<vi>, "UI.Refs.Controller"=w437:refnum<vi>)
            n168 = property class="Ring (strict)"(reference=w437, error in=w438) -> (error out=w439:errorcluster, "Strings []"=w443:string[], "Value"=w444:u16)  [unwired: 1 out]
            n169 = call "Get and Check PID Parameters.vi"("error in (no error)"=w439, "MulticolumnListbox in"=w436) -> ("error out"=w447:errorcluster, "PID Parameters"=w442:T16)  [unwired: 7 in, 1 out]
            n170 = Index Array(array=w443, index=w444) -> (element=w449:string)
            n171 = case shown="No Error" w447 {
              selector: w447 -> [_ w483]
              tunnel: w433 -> [w471 _]
              tunnel: w440 -> [w461 w485]
              tunnel: w449 -> [w456 _]
              tunnel: [w458 w485] -> w448
              tunnel: w446 -> [w467 w484]
              tunnel: [w464 w484] -> w445
              tunnel: w442 -> [w465 _]
              tunnel: [w450 w482] -> w441
              tunnel: w435 -> [w455 _]
              tunnel: w434 -> [w462 _]
              tunnel: w432 -> [w454 _]
              tunnel: w431 -> [w453 _]
              frame No Error {
                n172 = Bundle By Name(cluster=T13 {"Control Loop"="", "Gain Schedule"=[]} ("Parameters"), "Gain Schedule"=w465, "Control Loop"=w456) -> (w452:T13)
                n173 = call "Check Network Connection.vi"("IP Address"=w462, "CD Path"=w455, "connection info"=w471) -> ("error out"=w469:errorcluster, "connection info"=w470:T7)  [unwired: 7 in]
                n174 = Build Array (concatenate)(w467, "Tuning.Gains.UI.Update") -> (w464:string[])
                n175 = call "Update Configuration.vi"("error in (no error)"=w469, "Parameters"=w452, "connection info"=w470) -> ("error out"=w451:errorcluster, "Timed Out?"=w466:bool, "GetSettings"=w457:T2, "connection info"=w460:T7)  [unwired: 5 in]
                n176 = Bundle By Name(cluster=w461, "Settings"=w457) -> (w472:T1)
                n177 = case shown="False" w466 {
                  tunnel: w455 -> [w479 _]
                  tunnel: w454 -> [w477 _]
                  tunnel: w453 -> [w478 _]
                  tunnel: w452 -> [w475 _]
                  tunnel: w451 -> [w474 w480]
                  tunnel: [w473 w480] -> w450
                  frame False {
                    # "No timeout. Do nothing."
                    n178 = call "UI.Addon.Path.Parse.vi"("Cached Addon Path"=w479) -> ("Addon Name"=w476:string)  [unwired: 6 in, 4 out]
                    n179 = call "Update PID Parameters in System Definition.vi"("Name"=w476, "error in (no error)"=w474, "Parameters"=w475, "NIVS SysDefRoot Ref"=w477, "NIVS SysDef Ref"=w478) -> ("error out"=w473:errorcluster)  [unwired: 6 in]
                  }
                  frame True {
                    # "Handle timeout error."
                    n180 = One Button Dialog(message="The attempt to apply the PID settings failed.  Try reconnecting to the target by selecting File >> Configure and selecting the desired control add-on.") -> ()  [unwired: 1 in, 1 out]
                  }
                }
                n181 = Select(t=w461, s=w466, f=w472) -> (s? t:f=w459:T1)
                n182 = Bundle By Name(cluster=w459, "Comm Info"=w460) -> (w458:T1)
              }
              frame Error {
                n183 = call <vilib>:"Clear Errors.vi"("error in (no error)"=w483) -> ("error out"=w482:errorcluster)  [unwired: 5 in, 1 out]
              }
            }
          }
          frame "Tuning.Gains.Connect" {
            # "Request the current gains from the addon via custom device communication. Update UI as needed."
            n184 = Unbundle By Name(w494) -> ("Comm Info"=w486:T7, "CD IP"=w498:string, "CD Path"=w497:string)
            n185 = call "Check Network Connection.vi"("IP Address"=w497, "CD Path"=w498, "connection info"=w486) -> ("error out"=w496:errorcluster, "connection info"=w495:T7)  [unwired: 7 in]
            n186 = call "Get PID Configuration.vi"("error in (no error)"=w496, "connection info"=w495) -> ("Timed Out?"=w491:bool, "Settings"=w492:T2, "connection info"=w488:T7)  [unwired: 6 in, 1 out]
            n187 = case shown="False" w491 {
              tunnel: w494 -> [w505 w507]
              tunnel: [w504 w506] -> w493
              tunnel: w492 -> [w503 _]
              tunnel: w490 -> [w502 w510]
              tunnel: [w501 w510] -> w489
              tunnel: w488 -> [w500 w508]
              frame False {
                # "No timeout."
                n188 = Build Array (concatenate)(w502, string[] ["Tuning.UI.Enable", "Tuning.Gains.Menu.Enable", "Tuning.UI.Controllers.Update", "Tuning.Gains.UI.Update", "Controller.Connect"]) -> (w501:string[])
                n189 = Bundle By Name(cluster=w505, "Comm Info"=w500, "Settings"=w503) -> (w504:T1)
              }
              frame True {
                # "Timeout occurred."
                n190 = Bundle By Name(cluster=w507, "Comm Info"=w508) -> (w506:T1)
                n191 = One Button Dialog(message="The attempt to get the PID settings failed.  Try reconnecting to the target by selecting File >> Configure and selecting the desired control add-on.") -> ()  [unwired: 1 in, 1 out]
              }
            }
          }
          frame "Tuning.Gains.Menu.Disable" {
            # "Disable menu options. Mainly for when the system state is not connected."
            n192 = Unbundle By Name(w512) -> ("UI.PIDSettingsMenu"=w511:string[])
            n193 = Current VI's Menubar() -> (w515:refnum<k9>)
            n194 = for {
              tunnel: w515 -> [w521]
              tunnel: w511 -> [w519] mode=indexing
              shift-right: [w517] -> w513
              shift-left: w514 -> [w518]
              n195 = Set Menu Item Info(7:w519, 8:w518, 9:FALSE ("enabled"), 11:w521) -> (0:w517:errorcluster)  [unwired: 3 in, 1 out]
            }
          }
          frame "Tuning.Gains.Menu.Enable" {
            # "Enable menu options. System state is connected."
            n196 = Unbundle By Name(w525) -> ("UI.PIDSettingsMenu"=w524:string[])
            n197 = Current VI's Menubar() -> (w526:refnum<k9>)
            n198 = for {
              tunnel: w526 -> [w532]
              tunnel: w524 -> [w530] mode=indexing
              shift-right: [w528] -> w522
              shift-left: w523 -> [w529]
              n199 = Set Menu Item Info(7:w530, 8:w529, 9:TRUE ("enabled"), 11:w532) -> (0:w528:errorcluster)  [unwired: 3 in, 1 out]
            }
          }
          frame "Tuning.UI.Controllers.Update" {
            # "Update the list of valid PID controllers within the give addon."
            n200 = Unbundle By Name(w538) -> ("UI.Refs.Controller"=w534:refnum<vi>, "Settings.Control Loop Names"=w537:string[])
            n201 = property class="Ring (strict)"(reference=w534, error in=w536, "Strings []"=w537) -> (error out=w535:errorcluster)  [unwired: 1 out]
          }
          frame "Controller.Connect" {
            w545 = "/" ("string")
            # "#DLE - Need to use the controller here...."
            n202 = Unbundle By Name(w552) -> ("NIVS.SysDefRoot"=w565:refnum<k24>, "CD Path"=w540:string, "UI.Refs.Controller"=w550:refnum<vi>)
            n203 = global read "Constants.vi" "Name.PIDManualOutput"() -> (w553:string)
            n204 = global read "Constants.vi" "Name.ManualControl"() -> (w559:string)
            n205 = global read "Constants.vi" "Name.Channels"() -> (w564:string)
            n206 = property class="Ring (strict)"(reference=w550, error in=w548) -> (error out=w549:errorcluster, "Strings []"=w547:string[], "Value"=w546:u16)  [unwired: 1 out]
            n207 = call "UI.Addon.Path.Parse.vi"("Cached Addon Path"=w540) -> ("Addon Path"=w539:string)  [unwired: 6 in, 4 out]
            n208 = Index Array(array=w547, index=w546) -> (element=w544:string)
            n209 = global read "Constants.vi" "GUID.PIDController"() -> (w554:string)
            n210 = Concatenate Strings(w539, w545, w544) -> (w543:string)
            n211 = Concatenate Strings(w543, w545, w564, w545, w559) -> (w560:string)
            n212 = Concatenate Strings(w543, w545, w564, w545, w553) -> (w561:string)
            n213 = call "Get Dependent Nodes from SysDef Root.vi"("error in (no error)"=w549, "GUID"=w554, "Path"=w543, "SysDef Ref"=w565) -> ("error out"=w566:errorcluster, "Channels"=w541:string[], "Found"=w542:bool)  [unwired: 5 in]
            n214 = Index Array(array=w541, index=2) -> (element=w562:string)
            n215 = Build Array(w562, w560, w561) -> (w563:string[])
            n216 = Bundle By Name(cluster=w552, "Data.SlowChannels"=w563, "Data.UDPChannels"=w541, "Data.Found?"=w542) -> (w551:T1)
            n217 = case shown="True" w542 {
              tunnel: w555 -> [w567 w572]
              tunnel: [w567 w571] -> w556
              tunnel: w566 -> [w568 w569]
              tunnel: [w568 w569] -> w557
              frame False {
              }
              frame True {
                n218 = Build Array (concatenate)(w572, string[] ["Controller.UI.Update", "Controller.UI.Enable", "Controller.Acq.Start", "Controller.Channels.Get"]) -> (w571:string[])
              }
            }
          }
          frame "Controller.Acq.Start" {
            # "Do nothing."
            n219 = Unbundle By Name(w573) -> ("Data.UDPEngineQueue"=w576:refnum<queue>, "Data.UDPChannels"=w578:string[])
            n220 = Bundle By Name(cluster=T11 {"Action"=enum."Start Acq", "Channels"=[]}, "Channels"=w578) -> (w577:T11)
            n221 = Enqueue Element(queue=w576, element=w577, error in (no error)=w575) -> (error out=w574:errorcluster)  [unwired: 1 in, 2 out]
          }
          frame "Controller.Channels.Set" {
            # "Do nothing."
            n222 = Unbundle By Name(w581) -> ("Data.Found?"=w594:bool, "Addon.Connected?"=w591:bool, "Data.PreviousValues"=w592:dbl[], "Data.SlowChannels"=w590:string[], "NIVS.Workspace"=w597:T4)
            n223 = Boolean To (0,1)(Boolean="Manual Control") -> (0, 1=w595:i16)
            n224 = Build Array("Setpoint", w595, "Manual Output") -> (w589:dbl[])
            n225 = Not Equal?(x=w592, y=w589) -> (x != y?=w586:bool[])
            n226 = Compound Arithmetic op=AND(w594, w591) -> (w593:bool)
            n227 = case shown="True" w593 {
              tunnel: w586 -> [_ w608]
              tunnel: w589 -> [_ w607]
              tunnel: w583 -> [w601 w606]
              tunnel: [w601 w605] -> w584
              tunnel: w597 -> [w600 w604]
              tunnel: [w600 w603] -> w598
              tunnel: w590 -> [_ w602]
              frame False {
                # "Do nothing"
              }
              frame True {
                # "Connected & paths valid"
                n228 = for {
                  shift-right: [w614] -> w605
                  shift-left: w606 -> [w615]
                  shift-right: [w613] -> w603
                  shift-left: w604 -> [w612]
                  tunnel: w608 -> [w611] mode=indexing
                  tunnel: w607 -> [w610] mode=indexing
                  tunnel: w602 -> [w609] mode=indexing
                  n229 = case shown="True" w611 {
                    tunnel: w615 -> [w617 w623]
                    tunnel: [w617 w622] -> w614
                    tunnel: [w616 w621] -> w613
                    tunnel: w612 -> [w616 w620]
                    tunnel: w610 -> [_ w619]
                    tunnel: w609 -> [_ w618]
                    frame False {
                      # "Do nothing"
                    }
                    frame True {
                      # "Update channel"
                      n230 = call-poly <vilib>:"NI VeriStand - Set Channel Value.vi"("error in (no error)"=w623, "Value"=w619, "Channel"=w618, "WorkspaceManager in"=w620) -> ("error out"=w622:errorcluster, "WorkspaceManager out"=w621:T4)  [unwired: 6 in]
                    }
                  }
                }
              }
            }
            n231 = Bundle By Name(cluster=w581, "Data.PendingChange?"=FALSE ("Pending Change?"), "NIVS.Workspace"=w598) -> (w582:T1)
          }
          frame "Controller.Channels.Get" {
            # "Do nothing."
            n232 = Unbundle By Name(w625) -> ("Controller.SetpointRange.Max"=w633:dbl, "Controller.SetpointRange.Min"=w634:dbl, "Data.PendingChange?"=w632:bool, "Controller.OutputRange.Max"=w635:dbl, "Controller.OutputRange.Min"=w636:dbl, "Data.Found?"=w629:bool, "Addon.Connected?"=w628:bool, "NIVS.Workspace"=w630:T4, "Data.SlowChannels"=w631:string[])
            n233 = case shown="False" w632 {
              tunnel: w628 -> [w659 _]
              tunnel: w629 -> [w653 _]
              tunnel: w627 -> [w650 w669]
              tunnel: [w649 w669] -> w624
              tunnel: [w648 w670] -> w626
              tunnel: w630 -> [w647 _]
              tunnel: w631 -> [w645 _]
              tunnel: w625 -> [w644 w670]
              tunnel: w633 -> [w642 _]
              tunnel: w634 -> [w641 _]
              tunnel: w635 -> [w640 _]
              tunnel: w636 -> [w639 _]
              frame False {
                # "No pending data change.  Allow for a get."
                n234 = Compound Arithmetic op=AND(w653, w659) -> (w654:bool)
                n235 = case shown="True" w654 {
                  tunnel: w650 -> [w662 w668]
                  tunnel: [w662 w667] -> w649
                  tunnel: w647 -> [w661 w666]
                  tunnel: [w661 w665] -> w646
                  tunnel: w645 -> [_ w664]
                  tunnel: [dbl[] [0.0, 0.0, 0.0] ("Values") w663] -> w658
                  frame False {
                    # "Do Nothing."
                  }
                  frame True {
                    # "Connected & paths valid"
                    n236 = call-poly <vilib>:"NI VeriStand - Get Channel Value.vi"("error in (no error)"=w668, "Channels"=w664, "WorkspaceManager in"=w666) -> ("error out"=w667:errorcluster, "Values"=w663:dbl[], "WorkspaceManager out"=w665:T4)  [unwired: 6 in]
                  }
                }
                n237 = Index Array(array=w658) -> (element #1=w657:dbl, element #2=w652:dbl, element #3=w651:dbl)  [unwired: 3 in]
                n238 = To Long Integer(number=w652) -> (32bit integer=w656:i32)
                n239 = In Range and Coerce(upper limit=w642, x=w657, lower limit=w641) -> (coerced(x)=w643:dbl)  [unwired: 1 out]
                n240 = In Range and Coerce(upper limit=w640, x=w651, lower limit=w639) -> (coerced(x)=w638:dbl)  [unwired: 1 out]
                n241 = Not Equal To 0?(x=w656) -> (x != 0?=w655:bool)
                n242 = local write "Setpoint"(w643) -> ()
                n243 = local write "Manual Output"(w638) -> ()
                n244 = local write "Manual Control"(w655) -> ()
                n245 = Bundle By Name(cluster=w644, "NIVS.Workspace"=w646, "Data.PreviousValues"=w658) -> (w648:T1)
              }
              frame True {
                # "A change is pending.  Don't get channels as this would overwrite the pending change."
              }
            }
          }
          frame "Controller.UI.Initialize" {
            w685 = TRUE ("Manual Control")
            w686 = FALSE ("Manual Control")
            w684 = u8 2 ("X Scale.Scale Fit")
            # "Do nothing."
            n246 = Unbundle By Name(cluster{"Min":dbl, "Max":dbl} {"Min"=0.0, "Max"=0.0} ("input cluster")) -> ("Min"=w675:dbl, "Max"=w674:dbl)
            n247 = In Range and Coerce(upper limit=w674, x=0.0, lower limit=w675) -> (coerced(x)=w688:dbl)  [unwired: 1 out]
            n248 = property on="Setpoint" class="DigNum (strict)"(error in=w677, "Minimum"=w675, "Maximum"=w674, "Value"=w688) -> (error out=w690:errorcluster)  [unwired: 1 in, 1 out]
            n249 = local write "Manual Control"(w686) -> ()
            n250 = local write "Hold"(w686) -> ()
            n251 = local write "Autoscale X"(w685) -> ()
            n252 = local write "Autoscale Y"(w685) -> ()
            n253 = Bundle By Name(cluster=w679, "Data.Found?"=FALSE ("Controller.Selected?"), "Data.PendingChange?"=FALSE ("Pending Change?")) -> (w680:T1)
            n254 = In Range and Coerce(upper limit=w674, x=0.0, lower limit=w675) -> (coerced(x)=w681:dbl)  [unwired: 1 out]
            n255 = property on="Manual Output" class="DigNum (strict)"(error in=w690, "Minimum"=w675, "Maximum"=w674, "Value"=w681) -> (error out=w689:errorcluster)  [unwired: 1 in, 1 out]
            n256 = property on="Chart" class="WFChart (strict)"(error in=w689, "XScale.ScaleFit"=w684, "YScale.ScaleFit"=w684) -> (error out=w673:errorcluster)  [unwired: 1 in, 1 out]
            n257 = property on="Manual Control" class="Bool (strict)"(error in=w673, "Value"=FALSE ("Manual Control")) -> (error out=w672:errorcluster)  [unwired: 1 in, 1 out]
          }
          frame "Controller.UI.Update" {
            w712 = TRUE ("Manual Control")
            w713 = FALSE ("Manual Control")
            w711 = u8 2 ("X Scale.Scale Fit")
            # "Do nothing."
            n258 = Unbundle By Name(w702) -> ("NIVS.SysDefRoot"=w704:refnum<k24>, "CD Path"=w693:string, "UI.Refs.Controller"=w699:refnum<vi>)
            n259 = property class="Ring (strict)"(reference=w699, error in=w697) -> (error out=w698:errorcluster, "Strings []"=w700:string[], "Value"=w701:u16)  [unwired: 1 out]
            n260 = call "UI.Addon.Path.Parse.vi"("Cached Addon Path"=w693) -> ("Addon Path"=w692:string)  [unwired: 6 in, 4 out]
            n261 = Index Array(array=w700, index=w701) -> (element=w695:string)
            n262 = local write "Manual Control"(w713) -> ()
            n263 = local write "Hold"(w713) -> ()
            n264 = local write "Autoscale X"(w712) -> ()
            n265 = local write "Autoscale Y"(w712) -> ()
            n266 = Concatenate Strings(w692, "/" ("string"), w695) -> (w694:string)
            n267 = call "Get Controller Variables Ranges.vi"("error in (no error)"=w698, "Path"=w694, "NIVS.SysDef Ref"=w704) -> ("error out"=w722:errorcluster, "Setpoint Range"=w718:cluster{"Min":dbl, "Max":dbl}, "Output Range"=w719:cluster{"Min":dbl, "Max":dbl})  [unwired: 6 in]
            n268 = Unbundle By Name(w718) -> ("Min"=w716:dbl, "Max"=w717:dbl)
            n269 = Bundle By Name(cluster=w702, "Data.PendingChange?"=FALSE ("Pending Change?"), "Controller.SetpointRange"=w718, "Controller.OutputRange"=w719) -> (w703:T1)
            n270 = In Range and Coerce(upper limit=w717, x=0.0, lower limit=w716) -> (coerced(x)=w715:dbl)  [unwired: 1 out]
            n271 = property on="Setpoint" class="DigNum (strict)"(error in=w722, "Minimum"=w716, "Maximum"=w717, "Value"=w715) -> (error out=w721:errorcluster)  [unwired: 1 in, 1 out]
            n272 = Unbundle By Name(w719) -> ("Min"=w707:dbl, "Max"=w708:dbl)
            n273 = In Range and Coerce(upper limit=w708, x=0.0, lower limit=w707) -> (coerced(x)=w705:dbl)  [unwired: 1 out]
            n274 = property on="Manual Output" class="DigNum (strict)"(error in=w721, "Minimum"=w707, "Maximum"=w708, "Value"=w705) -> (error out=w720:errorcluster)  [unwired: 1 in, 1 out]
            n275 = property on="Chart" class="WFChart (strict)"(error in=w720, "XScale.ScaleFit"=w711, "YScale.ScaleFit"=w711) -> (error out=w709:errorcluster)  [unwired: 1 in, 1 out]
          }
          frame "Controller.UI.Enable" {
            n276 = Unbundle By Name(w724) -> ("UI.Chart.Refs"=w727:T10)
            n277 = call "UI Set DisableState.vi"("Enable?"=TRUE, "error in (no error)"=w729, "UI.Chart.Refs"=w727) -> ("error out"=w728:errorcluster, "UI.Chart.Refs"=w726:T10)  [unwired: 7 in]
            n278 = Bundle By Name(cluster=w724, "UI.Chart.Refs"=w726) -> (w725:T1)
          }
          frame "Controller.UI.Disable" {
            n279 = Unbundle By Name(w732) -> ("UI.Chart.Refs"=w735:T10)
            n280 = call "UI Set DisableState.vi"("Enable?"=FALSE, "error in (no error)"=w737, "UI.Chart.Refs"=w735) -> ("error out"=w736:errorcluster, "UI.Chart.Refs"=w734:T10)  [unwired: 7 in]
            n281 = Bundle By Name(cluster=w732, "UI.Chart.Refs"=w734) -> (w733:T1)
          }
          frame "Controller.UI.Buttons.Show" {
            w742 = TRUE ("Hold")
            # "Do nothing."
            n282 = property on="Apply Control Change" class="Bool"(error in=w741, "Visible"=w742) -> (error out=w743:errorcluster)  [unwired: 1 in, 1 out]
            n283 = property on="Revert Control Change" class="Bool"(error in=w743, "Visible"=w742) -> (error out=w740:errorcluster)  [unwired: 1 in, 1 out]
          }
          frame "Controller.UI.Buttons.Hide" {
            w750 = FALSE ("Hold")
            # "Do nothing."
            n284 = property on="Apply Control Change" class="Bool"(error in=w749, "Visible"=w750) -> (error out=w751:errorcluster)  [unwired: 1 in, 1 out]
            n285 = property on="Revert Control Change" class="Bool"(error in=w751, "Visible"=w750) -> (error out=w748:errorcluster)  [unwired: 1 in, 1 out]
            n286 = Bundle By Name(cluster=w752, "Data.PendingChange?"=FALSE) -> (w747:T1)
          }
          frame "Controller.Acq.Stop" {
            # "Do nothing."
            n287 = Unbundle By Name(w756) -> ("Data.UDPEngineQueue"=w759:refnum<queue>)
            n288 = Enqueue Element(queue=w759, element=T11 {"Action"=enum."Stop Acq", "Channels"=[]}, error in (no error)=w758) -> (error out=w757:errorcluster)  [unwired: 1 in, 2 out]
            n289 = Bundle By Name(cluster=w756, "Data.Found?"=FALSE ("Controller.Selected?")) -> (w755:T1)
          }
        }
      }
      frame Error {
        # "Error occurred. Display error to user. Then clear error and attempt to recover/continue."
        n290 = call <vilib>:"Simple Error Handler.vi"("error in (no error)"=w764) -> ("error out"=w763:errorcluster)  [unwired: 4 in, 4 out]
        n291 = call <vilib>:"Clear Errors.vi"("error in (no error)"=w763) -> ("error out"=w762:errorcluster)  [unwired: 5 in, 1 out]
      }
    }
  }
  n292 = while {
    tunnel: w18 -> [w769]
    tunnel: w17 -> [w774]
    tunnel: w19 -> [w770]
    tunnel: w11 -> [w768]
    stop <- w773 stop-if-true
    # "UDP Acq Loop"
    n293 = call "UDP Data Engine.vi"("WaveformChart Ref"=w770, "error in (no error)"=w768, "UDP Engine Queue"=w774, "WorkspaceManager"=w769) -> ("Exit"=w773:bool, "Update?"=w767:bool, "Waveform"=w771:waveform(dbl)[])  [unwired: 4 in, 1 out]
    n294 = case shown="False" w767 {
      tunnel: "Hold" -> [_ w776]
      tunnel: w771 -> [_ w775]
      frame False {
        # "Do Nothing."
      }
      frame True {
        # "Valid update."
        n295 = case shown="True" w776 {
          tunnel: w775 -> [w777 _]
          frame False {
            # "Update."
            "Chart" <- w777
          }
          frame True {
            # "Pause Updates"
          }
        }
      }
    }
  }
  n296 = Unbundle By Name(w29) -> ("NIVS.Workspace"=w28:T4, "NIVS.UserEvents"=w27:T14, "NIVS.SystemStateRefs"=w26:T6)
  n297 = flat-sequence {
    tunnel: w27 -> [w778]
    tunnel: w28 -> [w779]
    tunnel: w26 -> [w780]
    tunnel: [w780] -> w34
    tunnel: [w779] -> w33
    tunnel: [w781] -> w35
    tunnel: w34 -> [w782]
    tunnel: w33 -> [w781]
    tunnel: w35 -> [w783]
    frame #0 {
      n298 = Unregister For Events(event registration refnum=w778) -> ()  [unwired: 1 in, 1 out]
    }
    frame #1 {
      n299 = call <vilib>:"NI VeriStand - Close Engine State Change Notification.vi"("SystemStateRefs"=w782) -> ()  [unwired: 10 in, 1 out]
    }
    frame #2 {
      n300 = call <vilib>:"NI VeriStand - Close Workspace Manager Reference.vi"("WorkspaceManager"=w783) -> ()  [unwired: 10 in, 1 out]
    }
    frame #3 {
      n301 = invoke class="VI" method="FP.Close"() -> ()  [unwired: 3 in, 3 out]
    }
  }
